vi "freqout -- format.vi"(6 "Magn Field (T)":dbl, 7 "freqout action":enum16{"header", "one line", "one"}(ring)=enum."one line", 8 "segments string":string="Segments:{}", 9 "timestamp":timestamp, 10 "temperature":dbl, 11 "lorentzian":T1={"A (VHz)"=-1.0311345636926572, "ω (Hz)"=-1.0311345636926572, "Γ (Hz)"=-1.0311345636926572, "φ (rad)"=-1.0311345636926572, "Q"=-1.0311345636926572, "Norm  Ampl"=-1.0311345636926572, "z∞ (V)"=-1.0311345636926572+0.0i, "4corners"={"z (-pi/2)"=-1.0311345636926572+0.5736824521422934i, "z(inf)"=-0.5200164984937075+1.0975277942502903i, "z (pi/2)"=-1.0311345636926572+0.5736824521422934i, "z center"=-0.5136528600391839+0.580046090596817i, "z(0)"=-0.5200164984937075+1.0975277942502903i, "radius"=-1.0311345636926572}} {"z∞ (V)" format="%#_4p"; "Q" format="%#_4p"; "φ (rad)" format="%#_3p"; "Γ (Hz)" format="%#_5p"; "ω (Hz)" format="%#_9p"; "A (VHz)" format="%#_3p"}) -> (0 "output string":string)   [LabVIEW 2021]
uses:
  lorentzian.ctl
  circle corners.ctl
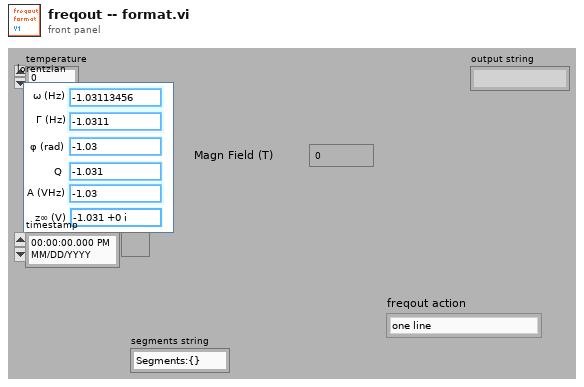
[diagram p1: front panel]
types:
  T1 = typedef "lorentzian.ctl" = cluster{"A (VHz)":dbl, "ω (Hz)":dbl, "Γ (Hz)":dbl, "φ (rad)":dbl, "Q":dbl, "Norm  Ampl":dbl, "z∞ (V)":cdb, "4corners":T2}
  T2 = typedef "circle corners.ctl" = cluster{"z (-pi/2)":cdb, "z(inf)":cdb, "z (pi/2)":cdb, "z center":cdb, "z(0)":cdb, "radius":dbl}
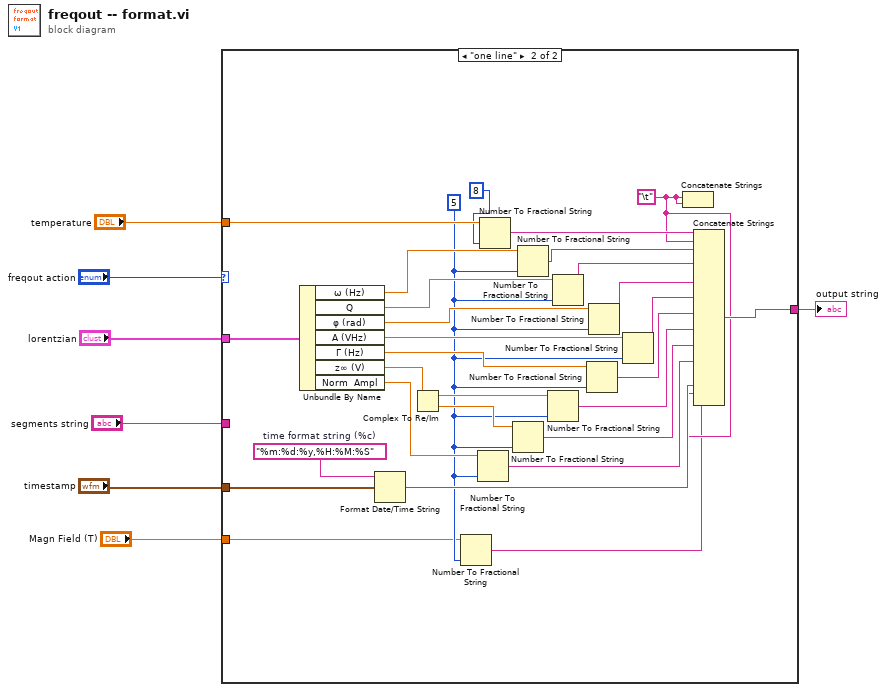
[diagram p0: block diagram]
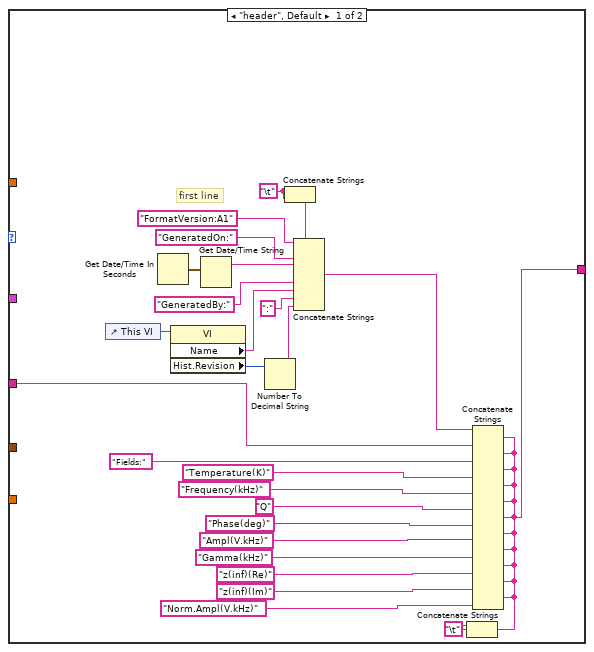
[diagram p2: hidden frame]
diagram:
  n1 = case shown="\"one line\"" "freqout action" {
    tunnel: [w9 w39] -> w2
    tunnel: "segments string" -> [w8 _]
    tunnel: "temperature" -> [_ w63]
    tunnel: "lorentzian" -> [_ w62]
    tunnel: "timestamp" -> [_ w61]
    tunnel: "Magn Field (T)" -> [_ w35]
    frame "header", Default {
      w20 = "\t"
      w29 = "\t"
      # "first line"
      n2 = control-ref of="This VI"() -> (w19:refnum<vi>)
      n3 = Get Date/Time In Seconds() -> (seconds since 1Jan1904=w24:timestamp)
      n4 = property class="VI"(reference=w19) -> ("Name"=w16:string, "Hist.Revision"=w18:u32)  [unwired: 1 in, 2 out]
      n5 = Get Date/Time String(seconds (now)=w24) -> (date string=w23:string)  [unwired: 2 in, 1 out]
      n6 = Number To Decimal String(number=w18) -> (decimal integer string=w14:string)  [unwired: 1 in]
      n7 = Concatenate Strings(w20, w20) -> (w15:string)
      n8 = Concatenate Strings("FormatVersion:A1", w15, "GeneratedOn:", w23, w15, "GeneratedBy:", w16, ":", w14) -> (w11:string)
      n9 = Concatenate Strings(w29, w29) -> (w10:string)
      n10 = Concatenate Strings(w11, w10, w8, w10, "Fields:", w10, "Temperature(K)", w10, "Frequency(kHz)", w10, "Q", w10, "Phase(deg)", w10, "Ampl(V.kHz)", w10, "Gamma(kHz)", w10, "z(inf)(Re)", w10, "z(inf)(Im)", w10, "Norm.Ampl(V.kHz)") -> (w9:string)
    }
    frame "one line" {
      w41 = "%m:%d:%y,%H:%M:%S"  # time format string (%c)
      w38 = "\t"
      w37 = i16 5 ("precision (6)")
      n11 = Unbundle By Name(w62) -> ("ω (Hz)"=w59:dbl, "Q"=w57:dbl, "φ (rad)"=w56:dbl, "A (VHz)"=w55:dbl, "Γ (Hz)"=w49:dbl, "z∞ (V)"=w45:cdb, "Norm  Ampl"=w44:dbl)
      n12 = Format Date/Time String(time format string (%c)=w41, seconds (now)=w61) -> (date/time string=w42:string)  [unwired: 1 in]
      n13 = Complex To Re/Im(x + iy=w45) -> (x=w43:dbl, y=w48:dbl)
      n14 = Number To Fractional String(number=w35, precision (6)=w37) -> (F-format string=w36:string)  [unwired: 2 in]
      n15 = Number To Fractional String(number=w44, precision (6)=w37) -> (F-format string=w46:string)  [unwired: 2 in]
      n16 = Number To Fractional String(number=w63, precision (6)=i16 8) -> (F-format string=w60:string)  [unwired: 2 in]
      n17 = Number To Fractional String(number=w48, precision (6)=w37) -> (F-format string=w47:string)  [unwired: 2 in]
      n18 = Number To Fractional String(number=w59, precision (6)=w37) -> (F-format string=w58:string)  [unwired: 2 in]
      n19 = Number To Fractional String(number=w43, precision (6)=w37) -> (F-format string=w50:string)  [unwired: 2 in]
      n20 = Number To Fractional String(number=w57, precision (6)=w37) -> (F-format string=w52:string)  [unwired: 2 in]
      n21 = Number To Fractional String(number=w49, precision (6)=w37) -> (F-format string=w51:string)  [unwired: 2 in]
      n22 = Number To Fractional String(number=w56, precision (6)=w37) -> (F-format string=w53:string)  [unwired: 2 in]
      n23 = Number To Fractional String(number=w55, precision (6)=w37) -> (F-format string=w54:string)  [unwired: 2 in]
      n24 = Concatenate Strings(w38, w38) -> ()  [unwired: 1 out]
      n25 = Concatenate Strings(w60, w38, w58, w38, w52, w38, w53, w38, w54, w38, w51, w38, w50, w38, w47, w38, w46, w38, w38, w42, w38, w36) -> (w39:string)
    }
  }
  "output string" <- w2
